vi "State Change Core.vi"(8 "error in (no error)":errorcluster, 10 "Transition State":refnum<class "State Pattern.lvclass">, 11 "State Pattern in":refnum<class "State Pattern.lvclass">) -> (0 "error out":errorcluster, 3 "State Pattern out":refnum<class "State Pattern.lvclass">)   [LabVIEW 2021, in "State Pattern.lvclass"]
uses:
  State Pattern.lvclass
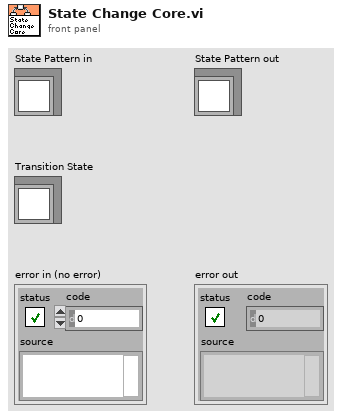
[diagram p1: front panel]
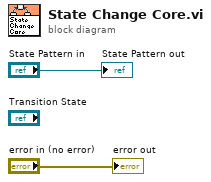
[diagram p0: block diagram]
diagram:
  "error out" <- "error in (no error)"
  "State Pattern out" <- "State Pattern in"
